vi "Finish.vi"   [LabVIEW 2018]
doc: "This VI is called just before exiting. It is expected to close I/O refnum, save collected data, etc."
uses:
  RefNums_DriverStation.vi
  RefNums_Actuators.vi
  RefNums_Sensors.vi
  <vilib>/Rock Robotics/WPI/Utilities/WPI_GetSetVariantRefNum.vi
types:
  T1 = typedef "WPI_MotorControlDeviceRef.ctl" = cluster{"DeviceStatus":errorcluster, "Type":T2, "PWM":cluster{"PWM Channel":T3, "DeadBand":T4}, "CAN":cluster{"Device Number":u8, "SetOutput VI Ref":variant, "GetOutput VI Ref":variant, "Enable VI Ref":variant, "Disable VI Ref":variant, "Data":variant}, "Invert":bool, "DIO PWM":cluster{"PWM \"Enable\" Channel":T3, "DIOChannel":T5, "PWM Rate":dbl}}
  T2 = typedef "WPI_MotorControlType.ctl" = enum16{"PWM", "CAN", "DIO PWM"}
  T3 = typedef "FPGA_DIOPWMChannel.ctl" = enum8{"PWM 0", "PWM 1", "PWM 2", "PWM 3", "PWM 4", "PWM 5", "PWM 6", "PWM 7", "PWM 8", "PWM 9", "PWM MXP 0", "PWM MXP 1", "PWM MXP 2", "PWM MXP 3", "PWM MXP 4", "PWM MXP 5", "PWM MXP 6", "PWM MXP 7", "PWM MXP 8", "PWM MXP 9", "Invalid"}
  T4 = typedef "WPI_PWMDeadband.ctl" = cluster{"Name":string, "maxPositivePwm":i32, "minPositivePwm":i32, "centerPwm":i32, "maxNegativePwm":i32, "minNegativePwm":i32, "angularRange":u16}
  T5 = typedef "FPGA_DIOChannel.ctl" = enum8{"DIO 0", "DIO 1", "DIO 2", "DIO 3", "DIO 4", "DIO 5", "DIO 6", "DIO 7", "DIO 8", "DIO 9", "DIO MXP 0", "DIO MXP 1", "DIO MXP 2", "DIO MXP 3", "DIO MXP 4", "DIO MXP 5", "DIO MXP 6", "DIO MXP 7", "DIO MXP 8", "DIO MXP 9", "DIO MXP 10", "DIO MXP 11", "DIO MXP 12", "DIO MXP 13", "DIO MXP 14", "DIO MXP 15", "SPI Port CS1", "SPI Port CS2", "SPI Port CS3", "SPI Port MISO", "SPI Port MOSI", "Invalid"}
  T6 = typedef "WPI_RobotDriveDevRef.ctl" = cluster{"DevStatus":errorcluster, "Motors[]":T1[], "Square Inputs":bool, "Max Output":dbl}
  T7 = typedef "WPI_AnalogChannelDevRef.ctl" = cluster{"DevStatus":errorcluster, "Analog Channel":T8}
  T8 = typedef "FPGA_AIChannel.ctl" = enum8{"AI 0", "AI 1", "AI 2", "AI 3", "AI MXP 0", "AI MXP 1", "AI MXP 2", "AI MXP 3", "Invalid"}
  T9 = typedef "WPI_SolenoidDevRef.ctl" = cluster{"DevStatus":errorcluster, "Pneumatics Control Module":u8, "Forward Solenoid Channel":T10, "Reverse Solenoid Channel":T10}
  T10 = typedef "WPI_SolenoidChannel.ctl" = enum8{"Solenoid 0", "Solenoid 1", "Solenoid 2", "Solenoid 3", "Solenoid 4", "Solenoid 5", "Solenoid 6", "Solenoid 7", "Invalid"}
  T11 = typedef "WPI_JoystickDevRef.ctl" = cluster{"Device":T12}
  T12 = typedef "WPI_JoystickDeviceEnum.ctl" = enum16{"USB 0", "USB 1", "USB 2", "USB 3", "USB 4", "USB 5"}
  T13 = typedef "WPI_CompressorDevRef.ctl" = cluster{"DevStatus":errorcluster, "Pneumatics Control Module":u8}
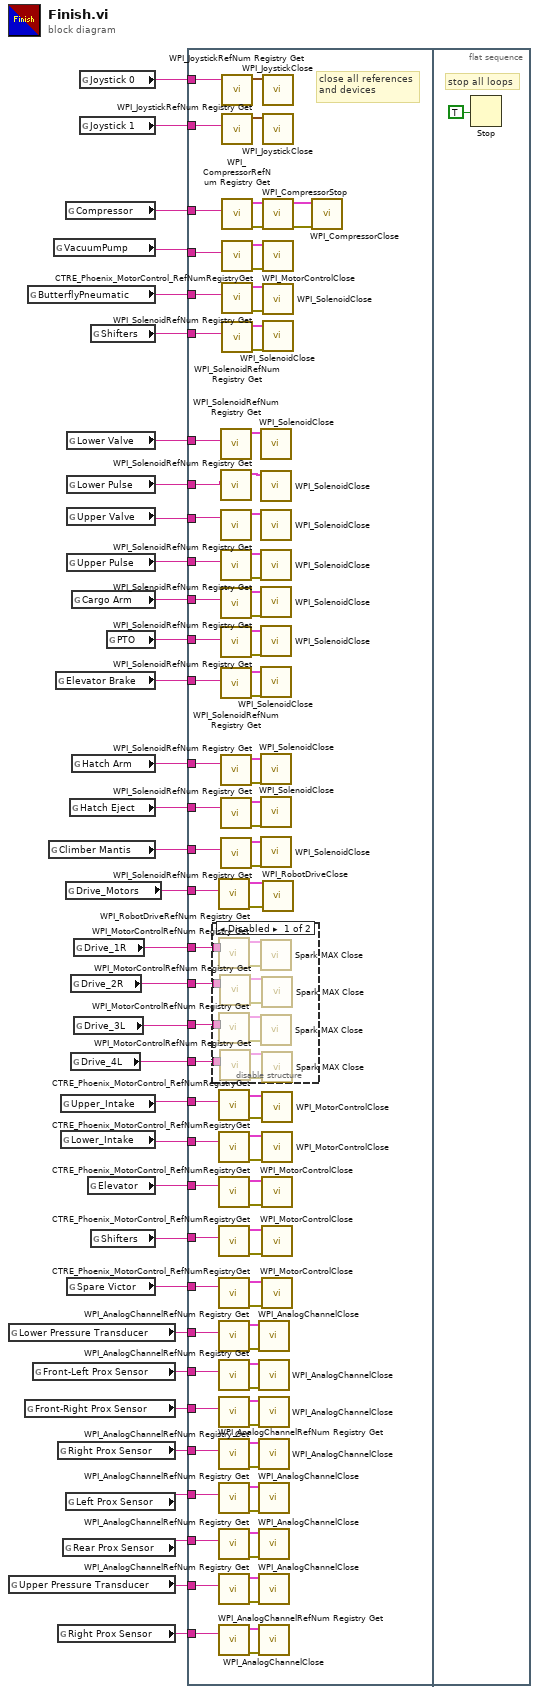
[diagram p0: block diagram]
diagram:
  n1 = global read "RefNums_Sensors.vi" "Lower Pressure Transducer"() -> (w7:string)
  n2 = global read "RefNums_Sensors.vi" "Upper Pressure Transducer"() -> (w21:string)
  n3 = global read "RefNums_Sensors.vi" "Front-Right Prox Sensor"() -> (w8:string)
  n4 = global read "RefNums_Actuators.vi" "ButterflyPneumatic"() -> (w31:string)
  n5 = global read "RefNums_Sensors.vi" "Front-Left Prox Sensor"() -> (w9:string)
  n6 = global read "RefNums_Actuators.vi" "Climber Mantis"() -> (w13:string)
  n7 = global read "RefNums_Actuators.vi" "VacuumPump"() -> (w29:string)
  n8 = global read "RefNums_Actuators.vi" "Elevator Brake"() -> (w16:string)
  n9 = global read "RefNums_Sensors.vi" "Right Prox Sensor"() -> (w23:string)
  n10 = global read "RefNums_Sensors.vi" "Right Prox Sensor"() -> (w6:string)
  n11 = global read "RefNums_Actuators.vi" "Upper_Intake"() -> (w26:string)
  n12 = global read "RefNums_Actuators.vi" "Lower_Intake"() -> (w25:string)
  n13 = global read "RefNums_Sensors.vi" "Rear Prox Sensor"() -> (w20:string)
  n14 = global read "RefNums_Actuators.vi" "Compressor"() -> (w32:string)
  n15 = global read "RefNums_Actuators.vi" "Drive_Motors"() -> (w1:string)
  n16 = global read "RefNums_Sensors.vi" "Left Prox Sensor"() -> (w22:string)
  n17 = global read "RefNums_Actuators.vi" "Lower Valve"() -> (w11:string)
  n18 = global read "RefNums_Actuators.vi" "Lower Pulse"() -> (w10:string)
  n19 = global read "RefNums_Actuators.vi" "Upper Valve"() -> (w12:string)
  n20 = global read "RefNums_Actuators.vi" "Upper Pulse"() -> (w28:string)
  n21 = global read "RefNums_Actuators.vi" "Spare Victor"() -> (w18:string)
  n22 = global read "RefNums_Actuators.vi" "Hatch Eject"() -> (w14:string)
  n23 = global read "RefNums_Actuators.vi" "Drive_2R"() -> (w4:string)
  n24 = global read "RefNums_Actuators.vi" "Drive_4L"() -> (w2:string)
  n25 = global read "RefNums_Actuators.vi" "Cargo Arm"() -> (w27:string)
  n26 = global read "RefNums_Actuators.vi" "Hatch Arm"() -> (w15:string)
  n27 = global read "RefNums_Actuators.vi" "Drive_1R"() -> (w5:string)
  n28 = global read "RefNums_Actuators.vi" "Drive_3L"() -> (w3:string)
  n29 = global read "RefNums_DriverStation.vi" "Joystick 0"() -> (w33:string)
  n30 = global read "RefNums_DriverStation.vi" "Joystick 1"() -> (w34:string)
  n31 = global read "RefNums_Actuators.vi" "Elevator"() -> (w24:string)
  n32 = global read "RefNums_Actuators.vi" "Shifters"() -> (w30:string)
  n33 = global read "RefNums_Actuators.vi" "Shifters"() -> (w19:string)
  n34 = global read "RefNums_Actuators.vi" "PTO"() -> (w17:string)
  n35 = flat-sequence {
    tunnel: w34 -> [w124]
    tunnel: w33 -> [w125]
    tunnel: w32 -> [w121]
    tunnel: w31 -> [w120]
    tunnel: w30 -> [w115]
    tunnel: w29 -> [w114]
    tunnel: w28 -> [w112]
    tunnel: w27 -> [w109]
    tunnel: w26 -> [w107]
    tunnel: w25 -> [w105]
    tunnel: w24 -> [w103]
    tunnel: w23 -> [w101]
    tunnel: w22 -> [w83]
    tunnel: w20 -> [w82]
    tunnel: w21 -> [w81]
    tunnel: w19 -> [w78]
    tunnel: w18 -> [w76]
    tunnel: w17 -> [w70]
    tunnel: w16 -> [w69]
    tunnel: w15 -> [w62]
    tunnel: w14 -> [w61]
    tunnel: w13 -> [w60]
    tunnel: w12 -> [w56]
    tunnel: w11 -> [w55]
    tunnel: w10 -> [w54]
    tunnel: w9 -> [w49]
    tunnel: w8 -> [w48]
    tunnel: w7 -> [w45]
    tunnel: w6 -> [w42]
    tunnel: w5 -> [w41]
    tunnel: w4 -> [w40]
    tunnel: w3 -> [w39]
    tunnel: w2 -> [w38]
    tunnel: w1 -> [w35]
    frame #0 {
      # "close all references\nand devices"
      n36 = disable-structure shown="Disabled" {
        disable-tunnel: w41 -> [w137 _]
        disable-tunnel: w40 -> [w132 _]
        disable-tunnel: w39 -> [w127 _]
        disable-tunnel: w38 -> [w126 _]
        frame Disabled {
          n37 = call <vilib>:"WPI_MotorControlRefNum Registry Get.vi"("refnum name"=w137) -> ("error out"=w136:errorcluster, "MotorControlDevRef"=w135:T1)  [unwired: 9 in]
          n38 = call <vilib>:"WPI_MotorControlRefNum Registry Get.vi"("refnum name"=w127) -> ("error out"=w129:errorcluster, "MotorControlDevRef"=w128:T1)  [unwired: 9 in]
          n39 = call <vilib>:"WPI_MotorControlRefNum Registry Get.vi"("refnum name"=w132) -> ("error out"=w134:errorcluster, "MotorControlDevRef"=w133:T1)  [unwired: 9 in]
          n40 = call <vilib>:"WPI_MotorControlRefNum Registry Get.vi"("refnum name"=w126) -> ("error out"=w130:errorcluster, "MotorControlDevRef"=w131:T1)  [unwired: 9 in]
          n41 = call <vilib>:"Spark MAX Close.vi"("error in"=w136, "MotorControlDeviceRef"=w135) -> ()  [unwired: 9 in, 1 out]
          n42 = call <vilib>:"Spark MAX Close.vi"("error in"=w129, "MotorControlDeviceRef"=w128) -> ()  [unwired: 9 in, 1 out]
          n43 = call <vilib>:"Spark MAX Close.vi"("error in"=w134, "MotorControlDeviceRef"=w133) -> ()  [unwired: 9 in, 1 out]
          n44 = call <vilib>:"Spark MAX Close.vi"("error in"=w130, "MotorControlDeviceRef"=w131) -> ()  [unwired: 9 in, 1 out]
        }
        frame Enabled {
        }
      }
      n45 = call <vilib>:"WPI_RobotDriveRefNum Registry Get.vi"("refnum name"=w35) -> ("error out"=w37:errorcluster, "RobotDriveDevRef"=w36:T6)  [unwired: 9 in]
      n46 = call <vilib>:"CTRE_Phoenix_MotorControl_RefNumRegistryGet.vi"("refnum name"=w107) -> ("error out"=w97:errorcluster, "PhoenixMotorControlDevRef"=w108:T1)  [unwired: 9 in]
      n47 = call <vilib>:"CTRE_Phoenix_MotorControl_RefNumRegistryGet.vi"("refnum name"=w105) -> ("error out"=w98:errorcluster, "PhoenixMotorControlDevRef"=w106:T1)  [unwired: 9 in]
      n48 = call <vilib>:"CTRE_Phoenix_MotorControl_RefNumRegistryGet.vi"("refnum name"=w103) -> ("error out"=w99:errorcluster, "PhoenixMotorControlDevRef"=w104:T1)  [unwired: 9 in]
      n49 = call <vilib>:"CTRE_Phoenix_MotorControl_RefNumRegistryGet.vi"("refnum name"=w78) -> ("error out"=w80:errorcluster, "PhoenixMotorControlDevRef"=w79:T1)  [unwired: 9 in]
      n50 = call <vilib>:"CTRE_Phoenix_MotorControl_RefNumRegistryGet.vi"("refnum name"=w76) -> ("error out"=w77:errorcluster, "PhoenixMotorControlDevRef"=w75:T1)  [unwired: 9 in]
      n51 = call <vilib>:"WPI_AnalogChannelRefNum Registry Get.vi"("refnum name"=w45) -> ("error out"=w46:errorcluster, "AIDeviceRef"=w47:T7)  [unwired: 9 in]
      n52 = call <vilib>:"WPI_AnalogChannelRefNum Registry Get.vi"("refnum name"=w49) -> ("error out"=w50:errorcluster, "AIDeviceRef"=w51:T7)  [unwired: 9 in]
      n53 = call <vilib>:"WPI_AnalogChannelRefNum Registry Get.vi"("refnum name"=w48) -> ("error out"=w52:errorcluster, "AIDeviceRef"=w53:T7)  [unwired: 9 in]
      n54 = call <vilib>:"WPI_AnalogChannelRefNum Registry Get.vi"("refnum name"=w101) -> ("error out"=w100:errorcluster, "AIDeviceRef"=w102:T7)  [unwired: 9 in]
      n55 = call <vilib>:"WPI_AnalogChannelRefNum Registry Get.vi"("refnum name"=w83) -> ("error out"=w88:errorcluster, "AIDeviceRef"=w89:T7)  [unwired: 9 in]
      n56 = call <vilib>:"WPI_AnalogChannelRefNum Registry Get.vi"("refnum name"=w82) -> ("error out"=w86:errorcluster, "AIDeviceRef"=w87:T7)  [unwired: 9 in]
      n57 = call <vilib>:"WPI_AnalogChannelRefNum Registry Get.vi"("refnum name"=w81) -> ("error out"=w84:errorcluster, "AIDeviceRef"=w85:T7)  [unwired: 9 in]
      n58 = call <vilib>:"WPI_AnalogChannelRefNum Registry Get.vi"("refnum name"=w42) -> ("error out"=w44:errorcluster, "AIDeviceRef"=w43:T7)  [unwired: 9 in]
      n59 = call <vilib>:"WPI_SolenoidRefNum Registry Get.vi"("refnum name"=w55) -> ("SolenoidDevRef"=w59:T9)  [unwired: 9 in, 1 out]
      n60 = call <vilib>:"WPI_SolenoidRefNum Registry Get.vi"("refnum name"=w54) -> ("SolenoidDevRef"=w58:T9)  [unwired: 9 in, 1 out]
      n61 = call <vilib>:"WPI_SolenoidRefNum Registry Get.vi"("refnum name"=w56) -> ("SolenoidDevRef"=w57:T9)  [unwired: 9 in, 1 out]
      n62 = call <vilib>:"WPI_SolenoidRefNum Registry Get.vi"("refnum name"=w112) -> ("error out"=w95:errorcluster, "SolenoidDevRef"=w111:T9)  [unwired: 9 in]
      n63 = call <vilib>:"WPI_SolenoidRefNum Registry Get.vi"("refnum name"=w109) -> ("error out"=w96:errorcluster, "SolenoidDevRef"=w110:T9)  [unwired: 9 in]
      n64 = call <vilib>:"WPI_SolenoidRefNum Registry Get.vi"("refnum name"=w70) -> ("error out"=w73:errorcluster, "SolenoidDevRef"=w74:T9)  [unwired: 9 in]
      n65 = call <vilib>:"WPI_SolenoidRefNum Registry Get.vi"("refnum name"=w69) -> ("error out"=w71:errorcluster, "SolenoidDevRef"=w72:T9)  [unwired: 9 in]
      n66 = call <vilib>:"WPI_SolenoidRefNum Registry Get.vi"("refnum name"=w62) -> ("error out"=w67:errorcluster, "SolenoidDevRef"=w68:T9)  [unwired: 9 in]
      n67 = call <vilib>:"WPI_SolenoidRefNum Registry Get.vi"("refnum name"=w61) -> ("error out"=w65:errorcluster, "SolenoidDevRef"=w66:T9)  [unwired: 9 in]
      n68 = call <vilib>:"WPI_SolenoidRefNum Registry Get.vi"("refnum name"=w60) -> ("error out"=w63:errorcluster, "SolenoidDevRef"=w64:T9)  [unwired: 9 in]
      n69 = call <vilib>:"WPI_JoystickRefNum Registry Get.vi"("refnum name"=w125) -> ("JoystickDevRef"=w122:T11)  [unwired: 9 in, 1 out]
      n70 = call <vilib>:"WPI_JoystickRefNum Registry Get.vi"("refnum name"=w124) -> ("JoystickDevRef"=w123:T11)  [unwired: 9 in, 1 out]
      n71 = call <vilib>:"WPI_CompressorRefNum Registry Get.vi"("refnum name"=w121) -> ("error out"=w91:errorcluster, "CompressorDevRef"=w118:T13)  [unwired: 9 in]
      n72 = call <vilib>:"CTRE_Phoenix_MotorControl_RefNumRegistryGet.vi"("refnum name"=w114) -> ("error out"=w92:errorcluster, "PhoenixMotorControlDevRef"=w113:T1)  [unwired: 9 in]
      n73 = call <vilib>:"WPI_SolenoidRefNum Registry Get.vi"("refnum name"=w120) -> ("error out"=w93:errorcluster, "SolenoidDevRef"=w119:T9)  [unwired: 9 in]
      n74 = call <vilib>:"WPI_SolenoidRefNum Registry Get.vi"("refnum name"=w115) -> ("error out"=w94:errorcluster, "SolenoidDevRef"=w116:T9)  [unwired: 9 in]
      n75 = call <vilib>:"WPI_AnalogChannelClose.vi"("error in (no error)"=w46, "AIDeviceRef"=w47) -> ()  [unwired: 9 in, 1 out]
      n76 = call <vilib>:"WPI_AnalogChannelClose.vi"("error in (no error)"=w50, "AIDeviceRef"=w51) -> ()  [unwired: 9 in, 1 out]
      n77 = call <vilib>:"WPI_AnalogChannelClose.vi"("error in (no error)"=w52, "AIDeviceRef"=w53) -> ()  [unwired: 9 in, 1 out]
      n78 = call <vilib>:"WPI_AnalogChannelClose.vi"("error in (no error)"=w100, "AIDeviceRef"=w102) -> ()  [unwired: 9 in, 1 out]
      n79 = call <vilib>:"WPI_AnalogChannelClose.vi"("error in (no error)"=w88, "AIDeviceRef"=w89) -> ()  [unwired: 9 in, 1 out]
      n80 = call <vilib>:"WPI_AnalogChannelClose.vi"("error in (no error)"=w86, "AIDeviceRef"=w87) -> ()  [unwired: 9 in, 1 out]
      n81 = call <vilib>:"WPI_AnalogChannelClose.vi"("error in (no error)"=w84, "AIDeviceRef"=w85) -> ()  [unwired: 9 in, 1 out]
      n82 = call <vilib>:"WPI_AnalogChannelClose.vi"("error in (no error)"=w44, "AIDeviceRef"=w43) -> ()  [unwired: 9 in, 1 out]
      n83 = call <vilib>:"WPI_SolenoidClose.vi"("SolenoidDevRef"=w59) -> ()  [unwired: 10 in, 1 out]
      n84 = call <vilib>:"WPI_SolenoidClose.vi"("SolenoidDevRef"=w58) -> ()  [unwired: 10 in, 1 out]
      n85 = call <vilib>:"WPI_SolenoidClose.vi"("SolenoidDevRef"=w57) -> ()  [unwired: 10 in, 1 out]
      n86 = call <vilib>:"WPI_SolenoidClose.vi"("error in (no error)"=w95, "SolenoidDevRef"=w111) -> ()  [unwired: 9 in, 1 out]
      n87 = call <vilib>:"WPI_SolenoidClose.vi"("error in (no error)"=w96, "SolenoidDevRef"=w110) -> ()  [unwired: 9 in, 1 out]
      n88 = call <vilib>:"WPI_SolenoidClose.vi"("error in (no error)"=w73, "SolenoidDevRef"=w74) -> ()  [unwired: 9 in, 1 out]
      n89 = call <vilib>:"WPI_SolenoidClose.vi"("error in (no error)"=w71, "SolenoidDevRef"=w72) -> ()  [unwired: 9 in, 1 out]
      n90 = call <vilib>:"WPI_SolenoidClose.vi"("error in (no error)"=w67, "SolenoidDevRef"=w68) -> ()  [unwired: 9 in, 1 out]
      n91 = call <vilib>:"WPI_SolenoidClose.vi"("error in (no error)"=w65, "SolenoidDevRef"=w66) -> ()  [unwired: 9 in, 1 out]
      n92 = call <vilib>:"WPI_SolenoidClose.vi"("error in (no error)"=w63, "SolenoidDevRef"=w64) -> ()  [unwired: 9 in, 1 out]
      n93 = call <vilib>:"WPI_MotorControlClose.vi"("error in"=w97, "MotorControlDevRef"=w108) -> ()  [unwired: 9 in, 1 out]
      n94 = call <vilib>:"WPI_MotorControlClose.vi"("error in"=w98, "MotorControlDevRef"=w106) -> ()  [unwired: 9 in, 1 out]
      n95 = call <vilib>:"WPI_MotorControlClose.vi"("error in"=w99, "MotorControlDevRef"=w104) -> ()  [unwired: 9 in, 1 out]
      n96 = call <vilib>:"WPI_MotorControlClose.vi"("error in"=w80, "MotorControlDevRef"=w79) -> ()  [unwired: 9 in, 1 out]
      n97 = call <vilib>:"WPI_MotorControlClose.vi"("error in"=w77, "MotorControlDevRef"=w75) -> ()  [unwired: 9 in, 1 out]
      n98 = call <vilib>:"WPI_JoystickClose.vi"("JoystickDevRef"=w122) -> ()  [unwired: 11 in]
      n99 = call <vilib>:"WPI_JoystickClose.vi"("JoystickDevRef"=w123) -> ()  [unwired: 11 in]
      n100 = call <vilib>:"WPI_CompressorStop.vi"("error in (no error)"=w91, "CompressorDevRef"=w118) -> ("error out"=w90:errorcluster, "CompressorDevRef"=w117:T13)  [unwired: 8 in]
      n101 = call <vilib>:"WPI_MotorControlClose.vi"("error in"=w92, "MotorControlDevRef"=w113) -> ()  [unwired: 9 in, 1 out]
      n102 = call <vilib>:"WPI_SolenoidClose.vi"("error in (no error)"=w93, "SolenoidDevRef"=w119) -> ()  [unwired: 9 in, 1 out]
      n103 = call <vilib>:"WPI_SolenoidClose.vi"("error in (no error)"=w94, "SolenoidDevRef"=w116) -> ()  [unwired: 9 in, 1 out]
      n104 = call <vilib>:"WPI_RobotDriveClose.vi"("error in (no error)"=w37, "RobotDriveDevRef"=w36) -> ()  [unwired: 9 in, 1 out]
      n105 = call <vilib>:"WPI_CompressorClose.vi"("error in (no error)"=w90, "CompressorDevRef"=w117) -> ()  [unwired: 9 in, 1 out]
    }
    frame #1 {
      # "stop all loops"
      n106 = Stop(stop? (T)=TRUE ("Quit")) -> ()
    }
  }
